vi "LVH5AreadWDTAttrs.vi"(8 "error in (no error)":errorcluster, 11 "Waveform Dataset Ref":T1) -> (0 "error out":errorcluster, 1 "dt":dbl, 2 "t0":timestamp, 3 "Waveform Dataset Ref out":T1)   [LabVIEW 2017]
uses:
  <vilib>/UPVI/lvhdf5/library.llb/HDF5 Ref.ctl
  <vilib>/UPVI/lvhdf5/attribute.llb/Simple H5Aread (Variant).vi
  <vilib>/UPVI/lvhdf5/attribute.llb/Simple H5Aread.xnode
panel:
  # "LVHDF5 Toolkit\nCopyright (c) 2005-2013 by Jason D. Sommerville\nCopyright (c) 2014 by UPVI, LLC.\n\nThis use and distribution of this file is governed by the terms found in \nLICENSE.txt distributed with this toolkit and installed at\n <user.lib>\\_lvhdf5\\LICENSE.txt"
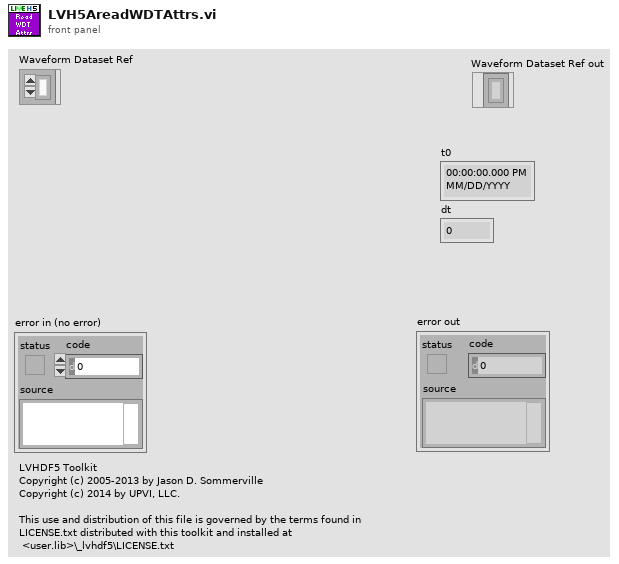
[diagram p1: front panel]
types:
  T1 = typedef "HDF5 Ref.ctl" = refnum<k1>
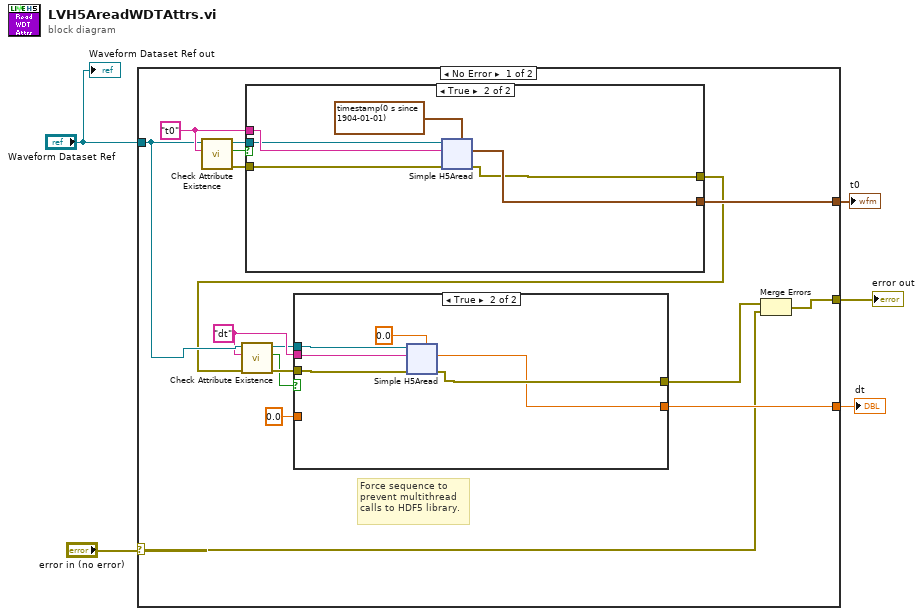
[diagram p0: block diagram]
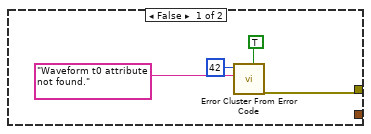
[diagram p3: hidden frame]
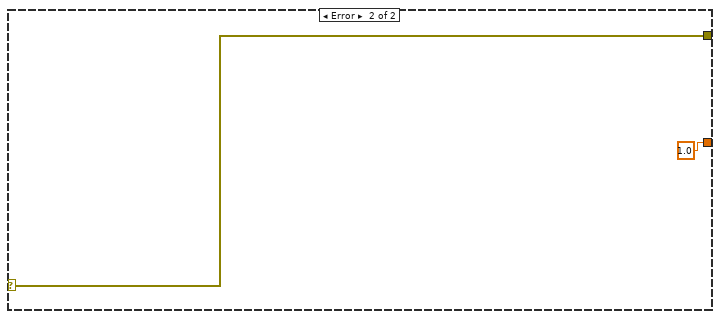
[diagram p4: hidden frame]
diagram:
  n1 = case shown="No Error" "error in (no error)" {
    selector: "error in (no error)" -> [w12 w91]
    tunnel: "Waveform Dataset Ref" -> [w16 _]
    tunnel: [w17 _] -> w2
    tunnel: [w14 w91] -> w1
    tunnel: [w13 1.0 ("Value")] -> w3
    frame No Error {
      w10 = "dt" ("name")
      w18 = "t0" ("name")
      # "Force sequence to\nprevent multithread\ncalls to HDF5 library."
      n2 = call <vilib>:"Check Attribute Existence.vi"("name"=w18, "HDF5 Ref"=w16) -> ("error out"=w19:errorcluster, "Exists"=w21:bool, "HDF5 Ref out"=w20:T1)  [unwired: 5 in]
      n3 = case shown="True" w21 {
        tunnel: w20 -> [_ w63]
        tunnel: w19 -> [_ w59]
        tunnel: w18 -> [_ w64]
        tunnel: [w56 w60] -> w6
        tunnel: [_ w61] -> w17
        frame False {
          n4 = call <vilib>:"Error Cluster From Error Code.vi"("is warning? (False)"=TRUE, "error message (\"\")"="Waveform t0 attribute not found." ("error message (\"\")"), "error code (0)"=42) -> ("error out"=w56:errorcluster)  [unwired: 6 in]
        }
        frame True {
          n5 = xnode "Simple H5Aread"("HDF5 Ref"=w63, "Name"=w64, "error in (no error)"=w59, "Type"=timestamp(0 s since 1904-01-01) ("Time Stamp")) -> ("error out"=w60:errorcluster, "Value"=w61:timestamp)  [unwired: 1 out]
        }
      }
      n6 = call <vilib>:"Check Attribute Existence.vi"("error in (no error)"=w6, "name"=w10, "HDF5 Ref"=w16) -> ("error out"=w9:errorcluster, "Exists"=w8:bool, "HDF5 Ref out"=w7:T1)  [unwired: 4 in]
      n7 = case shown="True" w8 {
        tunnel: [w23 w25] -> w15
        tunnel: 0.0 -> [w22 _]
        tunnel: w10 -> [_ w29]
        tunnel: w9 -> [w23 w28]
        tunnel: w7 -> [_ w27]
        tunnel: [w22 w24] -> w13
        frame False {
        }
        frame True {
          n8 = xnode "Simple H5Aread"("HDF5 Ref"=w27, "Name"=w29, "error in (no error)"=w28, "Type"=0.0) -> ("error out"=w25:errorcluster, "Value"=w24:dbl)  [unwired: 1 out]
        }
      }
      n9 = Merge Errors(w15, w12) -> (w14:errorcluster)
    }
    frame Error {
    }
  }
  "error out" <- w1
  "t0" <- w2
  "dt" <- w3
  "Waveform Dataset Ref out" <- "Waveform Dataset Ref"
